vi "Read Actions.vi"(8 "error in (no error)":errorcluster, 11 "lockin in":refnum<class "lockin.lvclass">) -> (0 "error out":errorcluster, 2 "Actions":T1, 3 "lockin out":refnum<class "lockin.lvclass">)   [LabVIEW 2016, in "lockin.lvclass"]
uses:
  lockin.lvclass
  Typedefs/lockin_actions.ctl
  lockin.lvclass/lockin.ctl
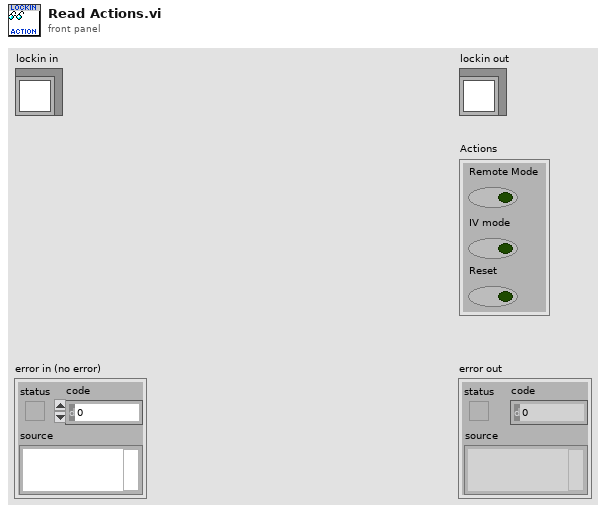
[diagram p1: front panel]
types:
  T1 = typedef "lockin.lvclass/lockin_actions.ctl" = cluster{"Remote Mode":bool, "IV mode":bool, "Reset":bool}
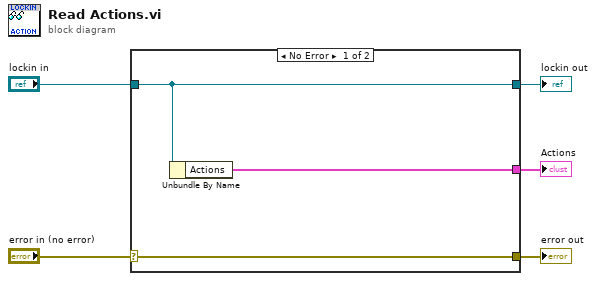
[diagram p0: block diagram]
diagram:
  n1 = case shown="No Error" "error in (no error)" {
    selector: "error in (no error)" -> [w8 w9]
    tunnel: [w8 w9] -> w4
    tunnel: [w7 w10] -> w2
    tunnel: "lockin in" -> [w7 w10]
    tunnel: [w6 _] -> w1
    frame No Error {
      n2 = Unbundle By Name(w7) -> ("Actions"=w6:T1)
    }
    frame Error {
    }
  }
  "error out" <- w4
  "lockin out" <- w2
  "Actions" <- w1
